vi "Get Sender.vi"(11 "Last Ack Msg Strategy in":refnum<class "Last Ack Msg Strategy.lvclass">) -> (2 "Sender":refnum<class "Sender.lvclass">)   [LabVIEW 2021, in "jettl.lvlib" / "Last Ack Msg Strategy.lvlib" / "Last Ack Msg Strategy.lvclass"]
uses:
  Last Ack Msg Strategy.lvclass
  Sender/Sender/Sender.lvclass
  Last Ack Msg Strategy.lvclass/Last Ack Msg Strategy.ctl
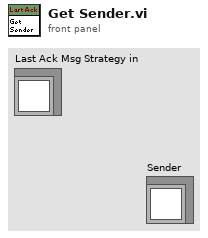
[diagram p1: front panel]
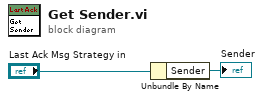
[diagram p0: block diagram]
diagram:
  n1 = Unbundle By Name("Last Ack Msg Strategy in") -> ("Sender"=→"Sender":refnum<class "Sender.lvclass">)
